vi "Waveform Write.vi"(8 "error in (no error)":errorcluster, 10 "Injection.Results":T1 {"Shots"."Results"."Off-Stage Avg Current" format="%#.6g"; "Shots"."Results"."Total Voltage Pulses" format="%#.6g"; "Shots"."Results"."Off-Stage Min Current" format="%#.6g"; "Shots"."Results"."Off-Stage Max Current" format="%#.6g"}, 11 "Parameters":T4={"Name"="", "Rate.Hz"=0, "Injectors.Count"=0, "Injector.Timeout"=0.0, "Injector.Timer"=[], "Injector.Info"=[], "Events.Count"=[], "Event.Parameters"={"Shots"=0, "Shot.InitialVoltage"=0.0, "Shot.Stages"=0, "Stages"=[{"Stage.Dwell.Level"=0.0, "PullIn.Type"=enum."Pull In Transition Dwells", "PullIn.Level"=0.0, "Transition.Type"=enum."Stage Transition Voltage Level", "Transition.Level"=0.0}]}, "DMA.Ref"=refnum, "Waveform.Refs"=[], "Waveform.Sessions"=[], "Waveform.Enable"=refnum, "FPGA.Status"=refnum, "Search.Data"=refnum, "Results.Data"=refnum, "Results.Values"=[], "Results.Selections"=[]}) -> (0 "error out":errorcluster, 2 "Injection.Results":T1 {"Shots"."Results"."Off-Stage Avg Current" format="%#.6g"; "Shots"."Results"."Total Voltage Pulses" format="%#.6g"; "Shots"."Results"."Off-Stage Min Current" format="%#.6g"; "Shots"."Results"."Off-Stage Max Current" format="%#.6g"}, 3 "Parameters":T4={"Name"="", "Rate.Hz"=0, "Injectors.Count"=0, "Injector.Timeout"=0.0, "Injector.Timer"=[], "Injector.Info"=[], "Events.Count"=[], "Event.Parameters"={"Shots"=0, "Shot.InitialVoltage"=0.0, "Shot.Stages"=0, "Stages"=[{"Stage.Dwell.Level"=0.0, "PullIn.Type"=enum."Pull In Transition Dwells", "PullIn.Level"=0.0, "Transition.Type"=enum."Stage Transition Voltage Level", "Transition.Level"=0.0}]}, "DMA.Ref"=refnum, "Waveform.Refs"=[], "Waveform.Sessions"=[], "Waveform.Enable"=refnum, "FPGA.Status"=refnum, "Search.Data"=refnum, "Results.Data"=refnum, "Results.Values"=[], "Results.Selections"=[]})   [LabVIEW 2015, in "Fuel Injection Addon Engine.lvlib"]
uses:
  Fuel Injection Addon Engine.lvlib
  Types/Async Parameters.ctl
  Shared/Types/Injector info.ctl
  Shared/Types/Shot.Parameters.ctl
  Shared/Types/Stage.Parameters.ctl
  Shared/Types/Stage.PullIn.Types.ctl
  Shared/Types/Stage.Transition.Types.ctl
  <vilib>/NI Veristand/Custom Device API/Waveform Data Reference.ctl
  <vilib>/NI VeriStand/Custom Device Waveform API/Single Waveform Write (DBL)/Single Waveform Write (DBL).lvclass
  <vilib>/NI/NIVS Inline Async API/_Data Access Engine/Data Access Engine/Types/Read.DVR.ctl
  <vilib>/NI/NIVS Inline Async API/_Data Access Engine/Access Type Classes/Read/Read.lvclass
  <vilib>/NI/NIVS Inline Async API/_Data Access Engine/Data Access Engine/Types/Write.DVR.ctl
  <vilib>/NI/NIVS Inline Async API/_Data Access Engine/Access Type Classes/Write/Write.lvclass
  Shared/Types/Analysis.Channels.Select.ctl
  Types/Injector Event Data Cluster.ctl
  RT Analysis/Controls/Shot Information Control.ctl
  Types/Stage.Measurements.ctl
  <vilib>/NI/NIVS Inline Async API/_Data Access Engine/Access Type Classes/Read/Read.lvclass/Read.ctl
  <vilib>/NI VeriStand/Custom Device Waveform API/Waveform Session.lvclass/Waveform Session.ctl
  <vilib>/NI VeriStand/Custom Device Waveform API/Single Waveform Write (DBL)/Single Waveform Write (DBL).lvclass/Single Waveform Write (DBL).ctl
  <vilib>/NI VeriStand/Custom Device Waveform API/Internal Comm Classes/WPL Comm/WPL Comm (1D DBL)/WPL Comm (1D DBL).lvclass/WPL Comm (1D DBL).ctl
  <vilib>/NI VeriStand/Custom Device Waveform API/Internal Comm Classes/WPL Comm/WPL Comm.lvclass/WPL Comm.ctl
  <vilib>/NI Veristand/Custom Device Waveform API/Single Waveform Write (DBL)/NI VeriStand - Write Single Waveform (DBL).vi
  <vilib>/NI/NIVS Inline Async API/_Data Access Engine/Data Access Engine/Methods/Read.Data.vi
  <vilib>/NI Veristand/Custom Device Waveform API/Internal Comm Classes/WPL Comm/WPL Comm (1D DBL)/Comm_write 1d dbl.vi
  <vilib>/NI Veristand/Custom Device Waveform API/Read Sample offset DVR.vi
  <vilib>/NI Veristand/Custom Device Waveform API/Check Opened.vi
  <vilib>/NI/NIVS Inline Async API/_Data Access Engine/Access Type Classes/Read/Read.ProcessData.vi
  <vilib>/NI Veristand/Custom Device Waveform API/Internal Comm Classes/WPL Comm/Direct Send WPL Command.vi
  <vilib>/NI Veristand/Custom Device Waveform API/Internal Comm Classes/WPL Comm/Convert Q Error to Shutdown Error.vi
  <vilib>/Utility/error.llb/Error Cluster From Error Code.vi
  <vilib>/NI Veristand/Custom Device Waveform API/NI_VS Custom Device Waveform API.lvlib
  <vilib>/NI/NIVS Inline Async API/_Data Access Engine/Data Access Engine/Data Access Engine.lvclass
  Shared/Fuel Injection Addon Shared.lvlib
  <vilib>/NI VeriStand/Custom Device API/Custom Device API.lvlib
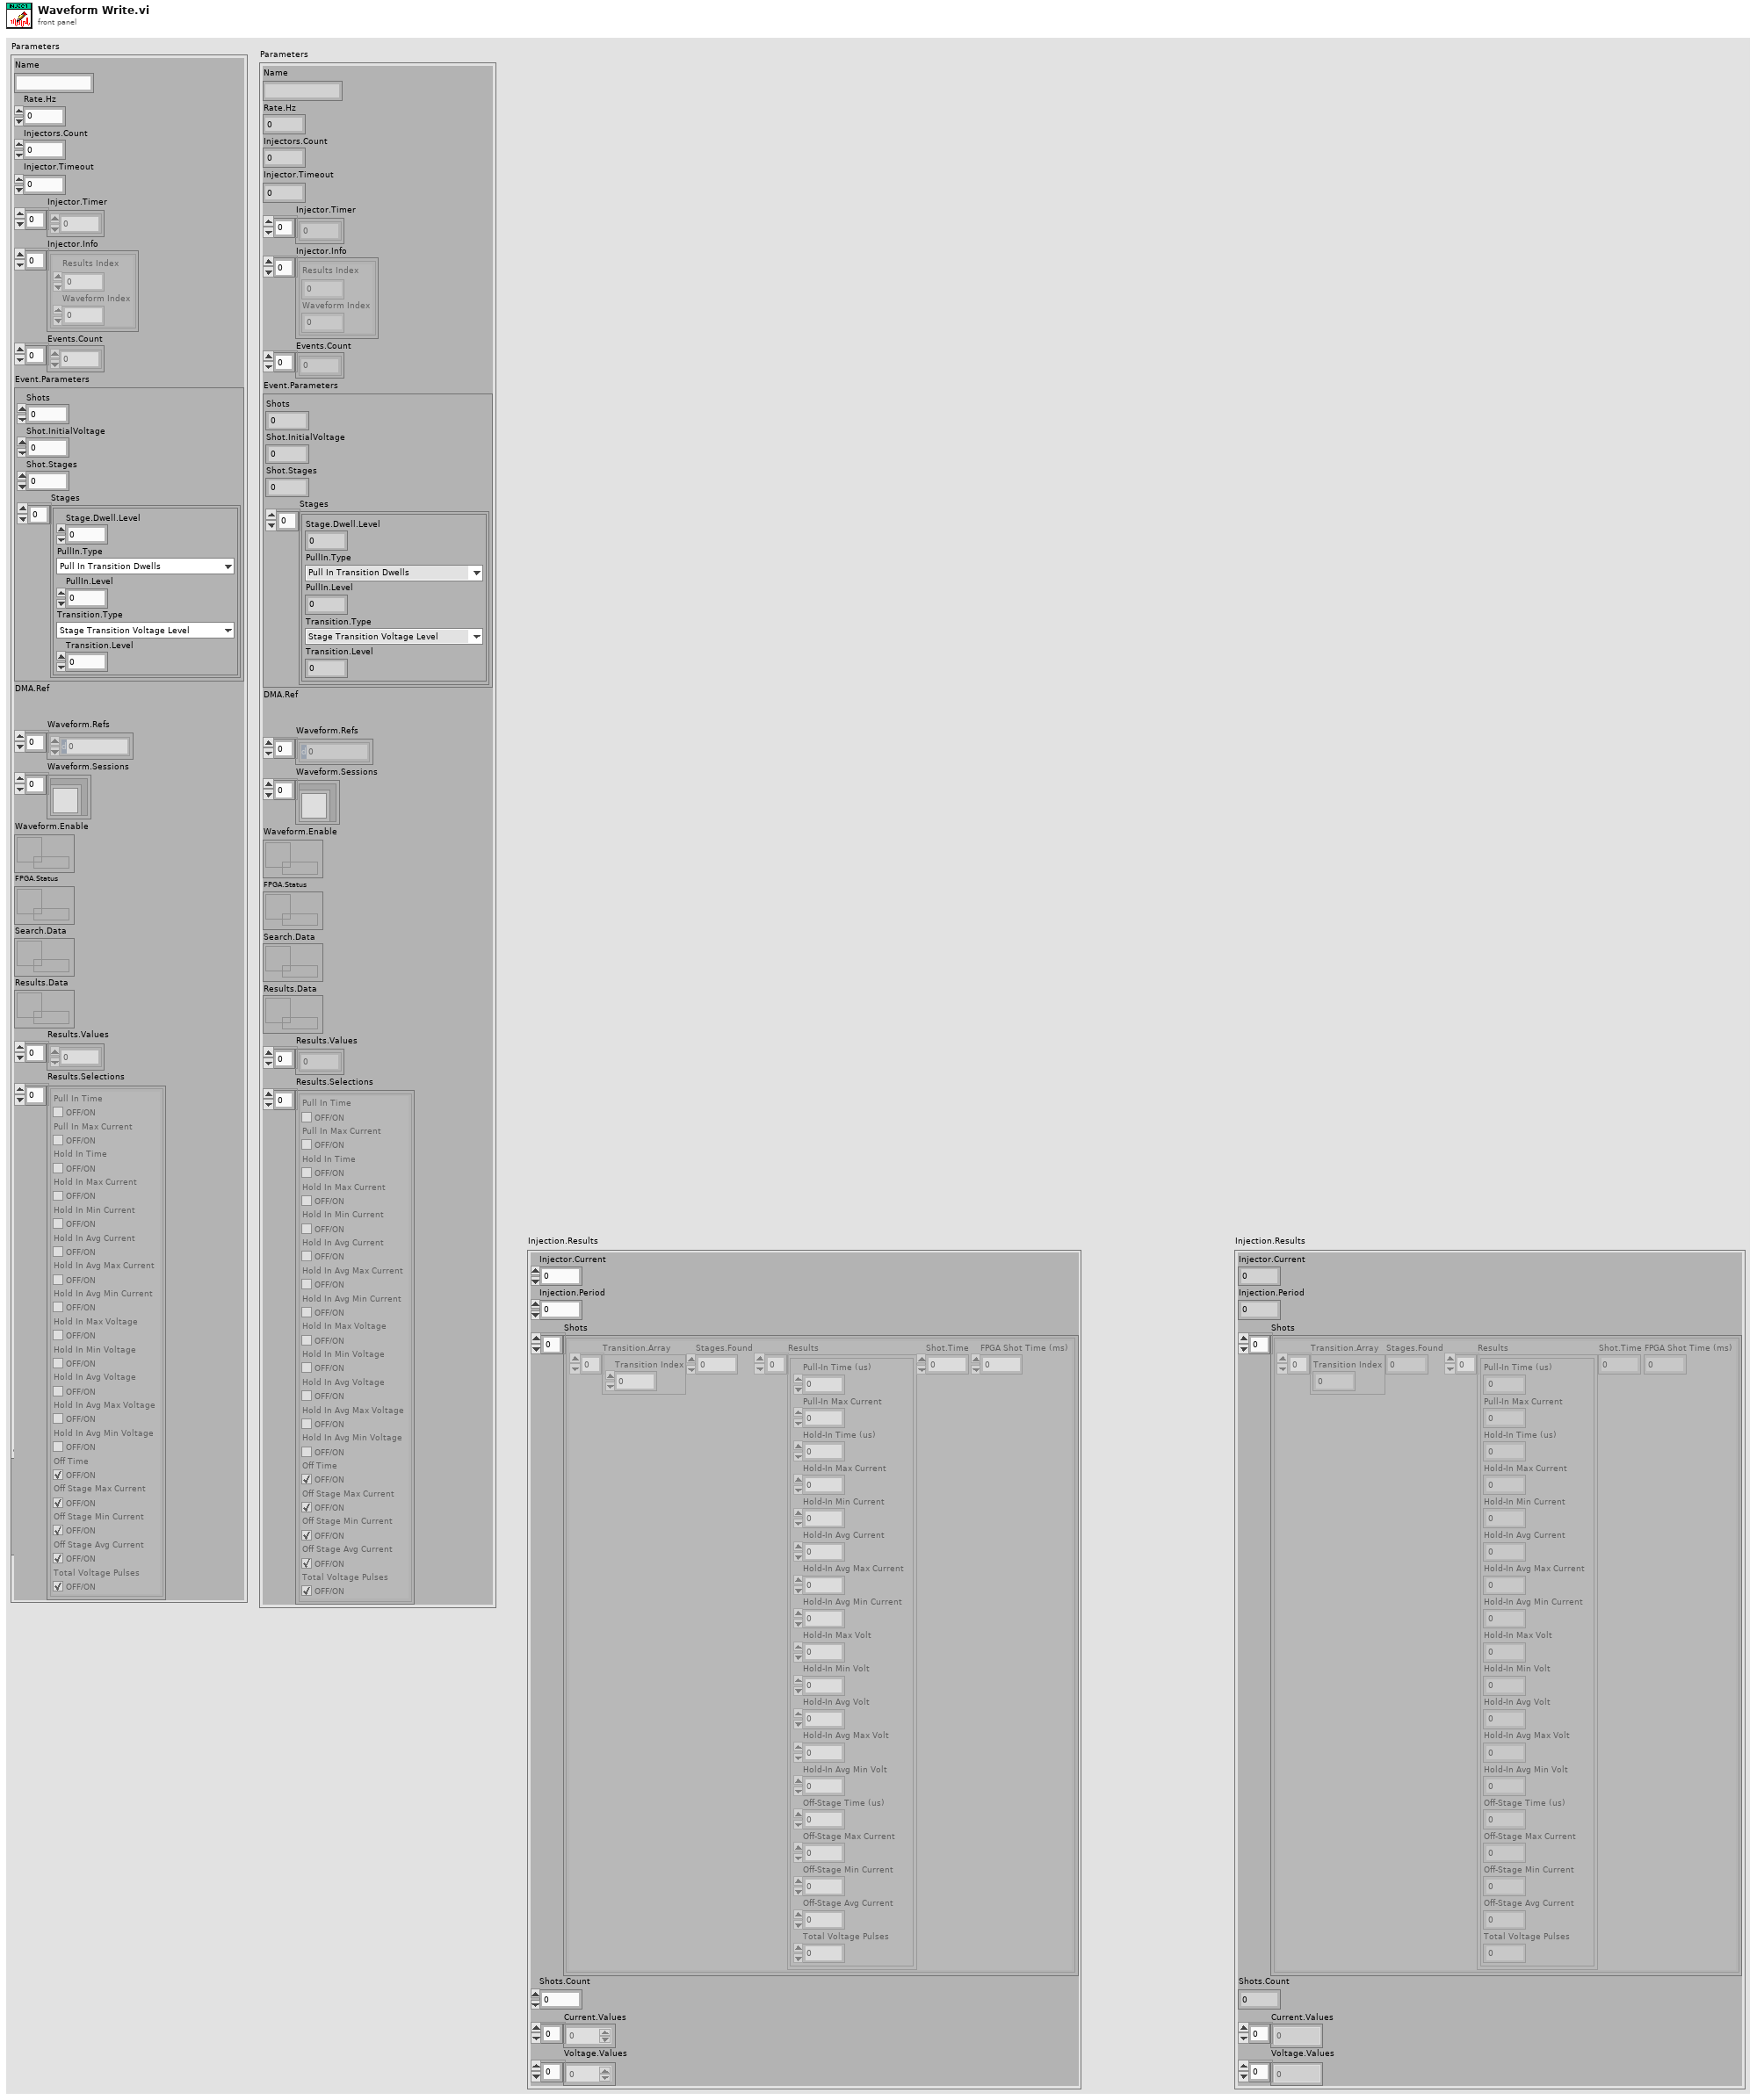
[diagram p1: front panel]
types:
  T1 = typedef "Fuel Injection Addon Engine.lvlib/Injector Event Data Cluster.ctl" = cluster{"Injector.Current":i16, "Injection.Period":dbl, "Shots":T2[], "Shots.Count":i32, "Current.Values":dbl[], "Voltage.Values":dbl[]}
  T2 = typedef "Fuel Injection Addon Engine.lvlib/Shot Information Control.ctl" = cluster{"Transition.Array":i32[], "Stages.Found":u16, "Results":T3[], "Shot.Time":dbl, "FPGA Shot Time (ms)":dbl}
  T3 = typedef "Fuel Injection Addon Engine.lvlib/Stage.Measurements.ctl" = cluster{"Pull-In Time (us)":dbl, "Pull-In Max Current":dbl, "Hold-In Time (us)":dbl, "Hold-In Max Current":dbl, "Hold-In Min Current":dbl, "Hold-In Avg Current":dbl, "Hold-In Avg Max Current":dbl, "Hold-In Avg Min Current":dbl, "Hold-In Max Volt":dbl, "Hold-In Min Volt":dbl, "Hold-In Avg Volt":dbl, "Hold-In Avg Max Volt":dbl, "Hold-In Avg Min Volt":dbl, "Off-Stage Time (us)":dbl, "Off-Stage Max Current":dbl, "Off-Stage Min Current":dbl, "Off-Stage Avg Current":dbl, "Total Voltage Pulses":dbl}
  T4 = typedef "Fuel Injection Addon Engine.lvlib/Async Parameters.ctl" = cluster{"Name":string, "Rate.Hz":u32, "Injectors.Count":u8, "Injector.Timeout":dbl, "Injector.Timer":u32[], "Injector.Info":T5[], "Events.Count":u64[], "Event.Parameters":T6, "DMA.Ref":refnum<k20>, "Waveform.Refs":T10[], "Waveform.Sessions":refnum<class "Single Waveform Write (DBL).lvclass">[], "Waveform.Enable":T11, "FPGA.Status":T12, "Search.Data":T11, "Results.Data":T12, "Results.Values":dbl[], "Results.Selections":T13[]}
  T5 = typedef "Fuel Injection Addon Shared.lvlib/Injector info.ctl" = cluster{"Results Index":i32, "Waveform Index":i32}
  T6 = typedef "Fuel Injection Addon Shared.lvlib/Shot.Parameters.ctl" = cluster{"Shots":u32, "Shot.InitialVoltage":dbl, "Shot.Stages":u32, "Stages":T7[]}
  T7 = typedef "Fuel Injection Addon Shared.lvlib/Stage.Parameters.ctl" = cluster{"Stage.Dwell.Level":dbl, "PullIn.Type":T8, "PullIn.Level":dbl, "Transition.Type":T9, "Transition.Level":dbl}
  T8 = typedef "Fuel Injection Addon Shared.lvlib/Stage.PullIn.Types.ctl" = enum8{"Pull In Transition Dwells", "Pull In Transition Current Drop"}
  T9 = typedef "Fuel Injection Addon Shared.lvlib/Stage.Transition.Types.ctl" = enum8{"Stage Transition Dwell Time", "Stage Transition Voltage Level", "Stage Transition Current Drop"}
  T10 = typedef "Custom Device API.lvlib/Waveform Data Reference.ctl" = i32
  T11 = typedef "Data Access Engine.lvlib/Data Access Engine.lvclass/Read.DVR.ctl" = refnum<data-value>
  T12 = typedef "Data Access Engine.lvlib/Data Access Engine.lvclass/Write.DVR.ctl" = refnum<data-value>
  T13 = typedef "Fuel Injection Addon Shared.lvlib/Analysis.Channels.Select.ctl" = cluster{"Pull In Time":bool, "Pull In Max Current":bool, "Hold In Time":bool, "Hold In Max Current":bool, "Hold In Min Current":bool, "Hold In Avg Current":bool, "Hold In Avg Max Current":bool, "Hold In Avg Min Current":bool, "Hold In Max Voltage":bool, "Hold In Min Voltage":bool, "Hold In Avg Voltage":bool, "Hold In Avg Max Voltage":bool, "Hold In Avg Min Voltage":bool, "Off Time":bool, "Off Stage Max Current":bool, "Off Stage Min Current":bool, "Off Stage Avg Current":bool, "Total Voltage Pulses":bool}
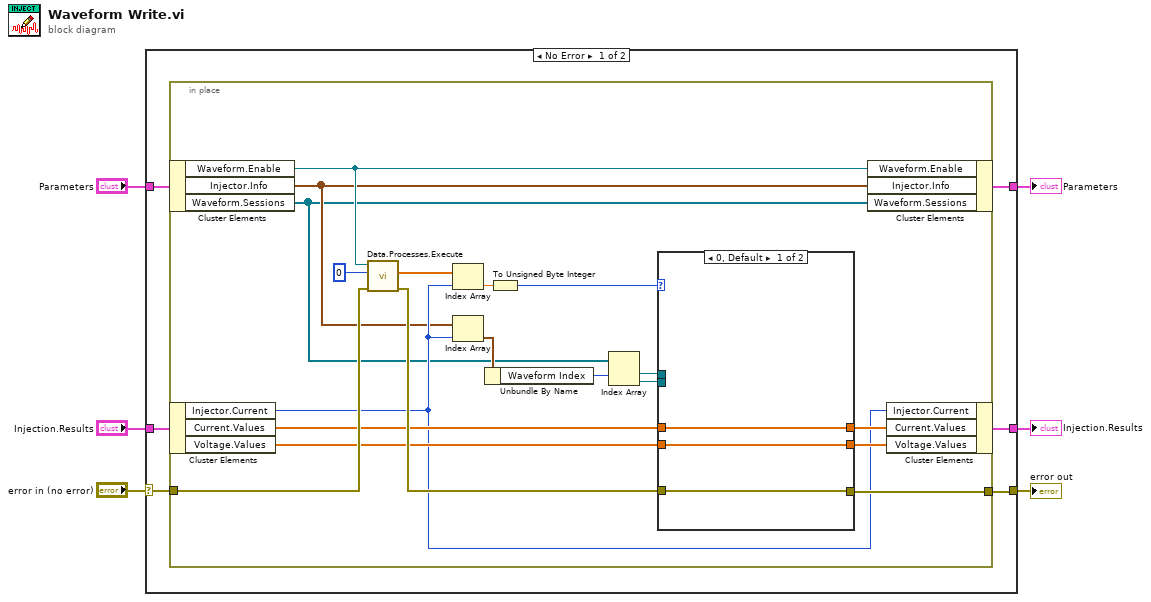
[diagram p0: block diagram]
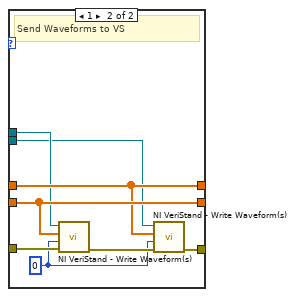
[diagram p2: hidden frame]
diagram:
  n1 = case shown="No Error" "error in (no error)" {
    selector: "error in (no error)" -> [w11 w45]
    tunnel: [w12 w45] -> w5
    tunnel: "Parameters" -> [w10 w44]
    tunnel: "Injection.Results" -> [w9 w43]
    tunnel: [w8 w44] -> w2
    tunnel: [w7 w43] -> w1
    frame No Error {
      n2 = in-place {
        in-place-border: [w31] -> w12
        in-place-border: w11 -> [w30]
        n3 = in-place-cluster #1(w10) -> ("Waveform.Enable"=w15:T11, "Injector.Info"=w14:T5[], "Waveform.Sessions"=w13:refnum<class "Single Waveform Write (DBL).lvclass">[])
        n4 = in-place-cluster #2(w9) -> ("Injector.Current"=w16:i16, "Current.Values"=w19:dbl[], "Voltage.Values"=w20:dbl[])
        n5 = call-poly <vilib>:"Data.Processes.Execute.vi"("error in (no error)"=w30, "timeout ms"=0 ("timeout in ms (0)"), "Ref"=w15) -> ("error out"=w29:errorcluster, "Values"=w28:dbl[])  [unwired: 6 in, 1 out]
        n6 = Index Array(array=w28, index=w16) -> (element=w27:dbl)
        n7 = Index Array(array=w14, index=w16) -> (element=w26:T5)
        n8 = Unbundle By Name(w26) -> ("Waveform Index"=w25:i32)
        n9 = To Unsigned Byte Integer(number=w27) -> (unsigned 8bit integer=w21:u8)
        n10 = Index Array(array=w13, index #1=w25) -> (element #1=w24:refnum<class "Single Waveform Write (DBL).lvclass">, element #2=w23:refnum<class "Single Waveform Write (DBL).lvclass">)  [unwired: 1 in]
        n11 = case shown="0, Default" w21 {
          tunnel: w20 -> [w33 w39]
          tunnel: w19 -> [w34 w38]
          tunnel: [w34 w38] -> w17
          tunnel: [w33 w39] -> w18
          tunnel: w29 -> [w32 w42]
          tunnel: [w32 w40] -> w31
          tunnel: w24 -> [_ w36]
          tunnel: w23 -> [_ w35]
          frame 0, Default {
          }
          frame 1 {
            w37 = 0 ("timeout in ms (0)")
            # "Send Waveforms to VS"
            n12 = call-poly <vilib>:"NI VeriStand - Write Waveform(s).vi"("error in (no error)"=w42, "timeout in ms (0)"=w37, "Data"=w39, "Single Waveform Write Session (DBL) in"=w36) -> ("error out"=w41:errorcluster)  [unwired: 5 in, 2 out]
            n13 = call-poly <vilib>:"NI VeriStand - Write Waveform(s).vi"("error in (no error)"=w41, "timeout in ms (0)"=w37, "Data"=w38, "Single Waveform Write Session (DBL) in"=w35) -> ("error out"=w40:errorcluster)  [unwired: 5 in, 2 out]
          }
        }
        n14 = in-place-cluster #1("Waveform.Enable"=w15, "Injector.Info"=w14, "Waveform.Sessions"=w13) -> (w8:T4)
        n15 = in-place-cluster #2("Injector.Current"=w16, "Current.Values"=w17, "Voltage.Values"=w18) -> (w7:T1)
      }
    }
    frame Error {
    }
  }
  "error out" <- w5
  "Parameters" <- w2
  "Injection.Results" <- w1
